vi "Filament switch.vi"(0 "Port Number":refnum<visa-resource-name>, 1 "Filament Switch":bool, 2 "error in (no error)":errorcluster) -> (3 "Status Byte":string, 4 "Filament Current (mA)":string, 5 "Timeout":bool, 6 "error out":errorcluster)   [LabVIEW 2019]
panel:
  out "Status":bool
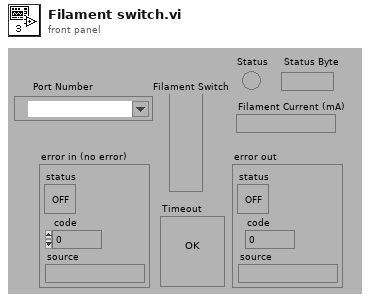
[diagram p1: front panel]
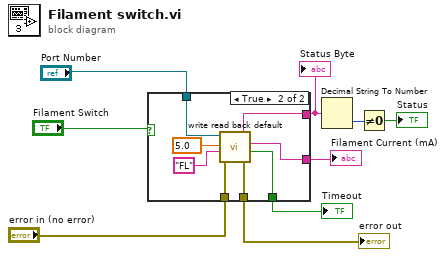
[diagram p0: block diagram]
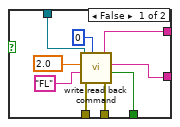
[diagram p2: hidden frame]
diagram:
  n1 = case shown="True" "Filament Switch" {
    tunnel: [w15 w24] -> w2
    tunnel: "error in (no error)" -> [w18 w23]
    tunnel: [w13 w22] -> w6
    tunnel: [w10 w21] -> w3
    tunnel: [w14 w20] -> w5
    tunnel: "Port Number" -> [w11 w19]
    frame False {
      n2 = call "write read back command.vi"("Input Parameter"=0, "error in (no error)"=w18, "Input Command"="FL", "Timeout Limit"=2.0, "Port Number"=w11) -> ("error out"=w13:errorcluster, "Timeout"=w14:bool, "Query Result"=w10:string, "Status Byte"=w15:string)  [unwired: 1 in]
    }
    frame True {
      n3 = call "write read back default.vi"("error in (no error)"=w23, "Input Command"="FL", "Timeout Limit"=5.0, "Port Number"=w19) -> ("error out"=w22:errorcluster, "Timeout"=w20:bool, "Query Result"=w21:string, "Status Byte"=w24:string)
    }
  }
  "error out" <- w6
  "Filament Current (mA)" <- w3
  "Timeout" <- w5
  "Status Byte" <- w2
  n4 = Decimal String To Number(string=w2) -> (number=w4:i32)  [unwired: 2 in, 1 out]
  n5 = Not Equal To 0?(x=w4) -> (x != 0?=→"Status":bool)
